vi "OSU_Connect.vi"(8 "error in (no error)":errorcluster, 10 "DeviceName":string, 11 ".NET Reference in":refnum<k24>) -> (0 "error out":errorcluster, 2 "ans":string, 3 "Reference out":refnum<k24>)   [LabVIEW 2017]
uses:
  LV_IL_Sample/DLL/InstrumentDLL.dll
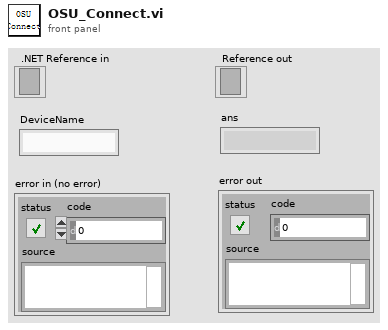
[diagram p1: front panel]
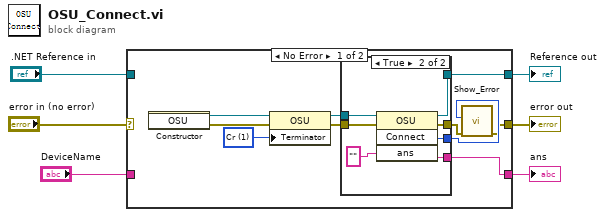
[diagram p0: block diagram]
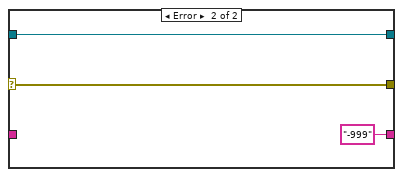
[diagram p3: hidden frame]
diagram:
  n1 = case shown="No Error" "error in (no error)" {
    selector: "error in (no error)" -> [_ w26]
    tunnel: "DeviceName" -> [_ _]
    tunnel: ".NET Reference in" -> [_ w25]
    tunnel: [w14 w25] -> w4
    tunnel: [w7 w26] -> w2
    tunnel: [w13 "-999" ("ans")] -> w1
    frame No Error {
      w10 = 1 items=["CrLf", "Cr", "Lf"] ("Terminator")
      n2 = constructor class="OSU"() -> (reference out=w12:refnum<k24>, error out=w11:errorcluster)  [unwired: 3 in, 1 out]
      n3 = property on="属性节点" class="OSU"(reference=w12, error in=w11, "Terminator"=w10) -> (reference out=w15:refnum<k24>, error out=w16:errorcluster)
      n4 = case shown="True" {
        selector: _ -> [_ _]
        tunnel: w16 -> [_ w23]
        tunnel: w15 -> [_ w22]
        tunnel: [_ w20] -> w14
        tunnel: [_ w19] -> w8
        tunnel: [_ w18] -> w9
        tunnel: [_ w17] -> w13
        frame False {
        }
        frame True {
          n5 = invoke on="调用节点" class="OSU" method="Connect"(reference=w22, error in=w23, "ans"="") -> (reference out=w20:refnum<k24>, error out=w18:errorcluster, "Connect"=w19:i32, "ans"=w17:string)  [unwired: 1 in]
        }
      }
      n6 = call "Show_Error.vi"("error in (no error)"=w9, "Error"=w8) -> ("error out"=w7:errorcluster)  [unwired: 9 in]
    }
    frame Error {
    }
  }
  "error out" <- w2
  "Reference out" <- w4
  "ans" <- w1
